vi "IMAQController.OverlayImage.vi"(0 "Image In":T2, 3 "Color":u32(colorbox)=16711680, 5 "error in":errorcluster, 9 "Overlay Lines":T1(array[cluster])) -> (14 "Image Out":T2, 19 "error out":errorcluster)   [LabVIEW 2014, in "IMAQController.lvlib"]
uses:
  IMAQController.lvlib
  <vilib>/vision/Image Controls.llb/IMAQ Image.ctl
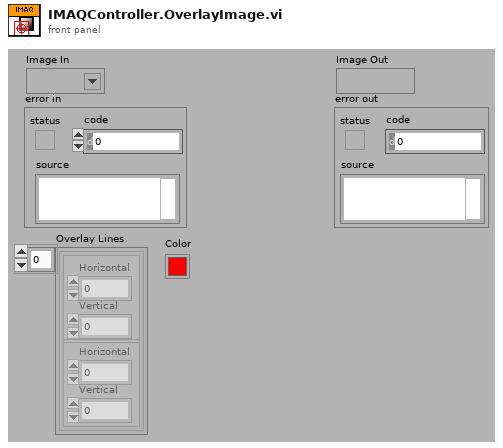
[diagram p1: front panel]
types:
  T1 = cluster{cluster{"Horizontal":i32, "Vertical":i32}, cluster{"Horizontal":i32, "Vertical":i32}}[]
  T2 = typedef "IMAQ Image.ctl" = refnum<image>
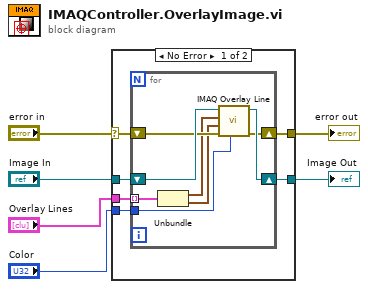
[diagram p0: block diagram]
diagram:
  n1 = case shown="No Error" "error in" {
    selector: "error in" -> [w11 w22]
    tunnel: [w8 w22] -> w5
    tunnel: "Image In" -> [w12 w21]
    tunnel: [w7 w21] -> w3
    tunnel: "Overlay Lines" -> [w10 _]
    tunnel: "Color" -> [w9 _]
    frame No Error {
      n2 = for {
        shift-right: [w19] -> w7
        shift-left: w12 -> [w20]
        shift-right: [w17] -> w8
        shift-left: w11 -> [w18]
        tunnel: w10 -> [w16] mode=indexing
        tunnel: w9 -> [w13]
        n3 = Unbundle(w16) -> (w14:cluster{"Horizontal":i32, "Vertical":i32}, w15:cluster{"Horizontal":i32, "Vertical":i32})
        n4 = call "IMAQ Overlay Line"("Color"=w13, "error in (no error)"=w18, "End Point"=w15, "Start Point"=w14, "Image"=w20) -> ("error out"=w17:errorcluster, "Image Out"=w19:T2)  [unwired: 5 in]
      }
    }
    frame Error {
    }
  }
  "Image Out" <- w3
  "error out" <- w5
